vi "ActiveX_test.vi"() -> ()   [LabVIEW 2011]
panel:
  out "Connected":bool
  in  "conn":bool
  out "error out":errorcluster
  in  "stop":bool
  out "DEC(sec)":dbl format="%<%H:%M:%S>t"
  out "RA(sec)":dbl format="%<%H:%M:%S%1u>t"
  in  "Output EPOCH":dbl
  in  "ScopeSim._Telescope":refnum<k7>
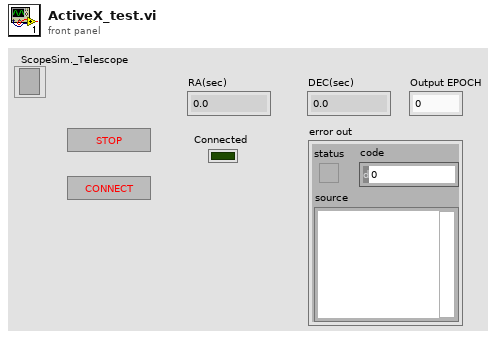
[diagram p1: front panel]
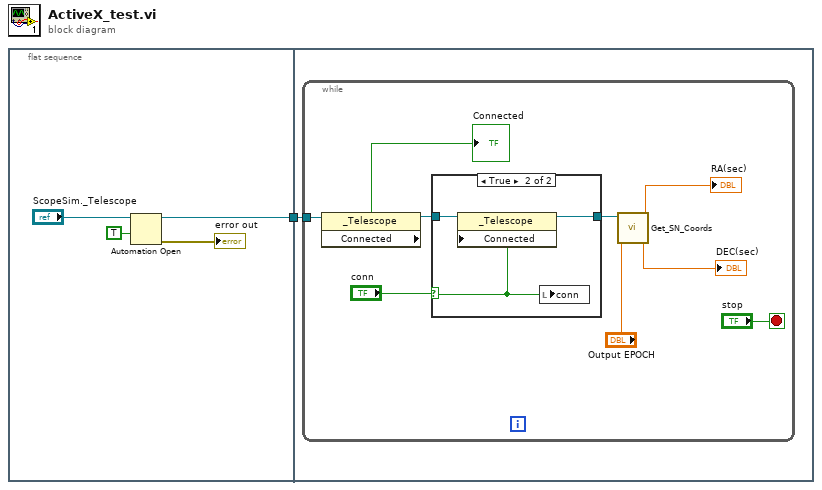
[diagram p0: block diagram]
diagram:
  n1 = flat-sequence {
    tunnel: [w3] -> w1
    tunnel: w1 -> [w6]
    frame #0 {
      n2 = Automation Open(Automation Refnum="ScopeSim._Telescope", 9:TRUE ("open new instance (false)")) -> (Automation Refnum=w3:refnum<k7>, error out=→"error out":errorcluster)  [unwired: 2 in]
    }
    frame #1 {
      n3 = while {
        tunnel: w6 -> [w11]
        stop <- "stop" stop-if-true
        n4 = property class="_Telescope"(reference=w11) -> (reference out=w9:refnum<k7>, "Connected"=→"Connected":bool)  [unwired: 1 in, 1 out]
        n5 = case shown="True" "conn" {
          selector: "conn" -> [_ w17]
          tunnel: w9 -> [w16 w19]
          tunnel: [w16 w18] -> w8
          frame False {
          }
          frame True {
            n6 = property class="_Telescope"(reference=w19, "Connected"=w17) -> (reference out=w18:refnum<k7>)  [unwired: 1 in, 1 out]
            n7 = local write "conn"(w17) -> ()
          }
        }
        n8 = call "Get_SN_Coords.vi"("Output EPOCH"="Output EPOCH", "ScopeSim._Telescope"=w8) -> ("DEC(sec)"=→"DEC(sec)":dbl, "RA(sec)"=→"RA(sec)":dbl)  [unwired: 8 in]
      }
    }
  }
